vi "Wrapper.vi"(8 "error in (no error)":errorcluster, 10 "Actor in":refnum<class "Actor.lvclass">, 11 "Change Heater Ctl Params in":refnum<class "Change Heater Ctl Params.lvclass">) -> (0 "error out":errorcluster, 3 "Actor out":refnum<class "Actor.lvclass">)   [LabVIEW 2017, in "Controller.lvlib" / "Change Heater Ctl Params.lvclass"]
uses:
  Change Heater Ctl Params.lvclass
  <vilib>/ActorFramework/Actor/Actor.lvclass
  Change Heater Ctl Params.lvclass/Change Heater Ctl Params.ctl
  gController.lvclass
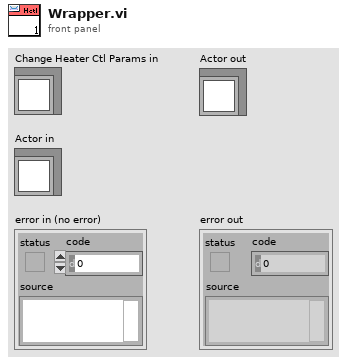
[diagram p1: front panel]
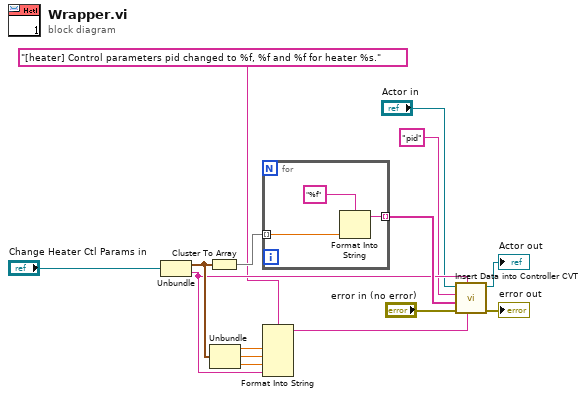
[diagram p0: block diagram]
diagram:
  n1 = Unbundle("Change Heater Ctl Params in") -> (w13:cluster{"p":dbl, "i":dbl, "d":dbl}, w12:string)
  n2 = Cluster To Array(cluster=w13) -> (array=w14:dbl[])
  n3 = Unbundle(w13) -> ("p"=w8:dbl, "i"=w9:dbl, "d"=w10:dbl)
  n4 = for {
    tunnel: w14 -> [w18] mode=indexing
    tunnel: [w16] -> w15 mode=indexing
    n5 = Format Into String(format string="%f", w18) -> (resulting string=w16:string)  [unwired: 2 in, 1 out]
  }
  n6 = Format Into String(format string="[heater] Control parameters pid changed to %f, %f and %f for heater %s.", w8, w9, w10, w12) -> (resulting string=w11:string)  [unwired: 2 in, 1 out]
  n7 = call "Insert Data into Controller CVT.vi"("Update MSG"=w11, "Group"=w12, "error in"="error in (no error)", "Data"=w15, "tag"="pid", "Actor in"="Actor in") -> ("error out"=→"error out":errorcluster, "Actor Out"=→"Actor out":refnum<class "Actor.lvclass">)  [unwired: 4 in]
